vi "judgeExtremeType.vi"(9 "next":i8, 10 "current":i8, 11 "previous":i8) -> (0 "isExtreme?":bool, 3 "extreme Type":u8)   [LabVIEW 2016]
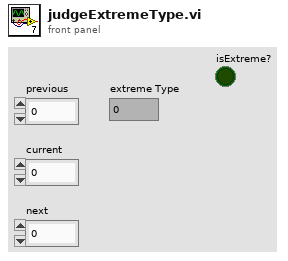
[diagram p1: front panel]
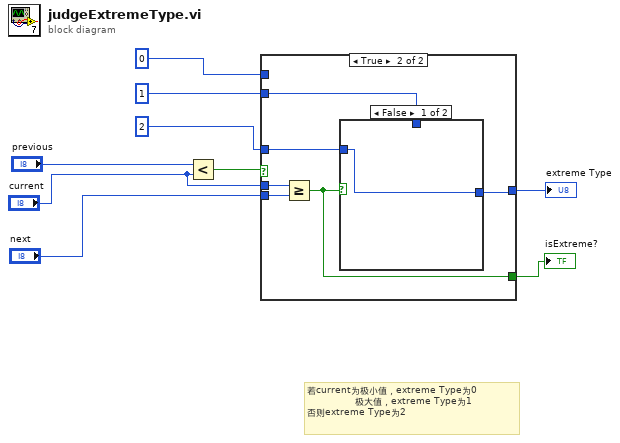
[diagram p0: block diagram]
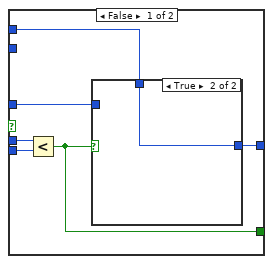
[diagram p2: hidden frame]
diagram:
  # "若current为极小值，extreme Type为0\n                极大值，extreme Type为1\n否则extreme Type为2"
  n1 = Less?(x="previous", y="current") -> (x < y?=w6:bool)
  n2 = case shown="True" w6 {
    tunnel: "current" -> [w15 w23]
    tunnel: "next" -> [w14 w22]
    tunnel: [w12 w19] -> w9
    tunnel: i16 1 -> [_ w21]
    tunnel: i16 0 -> [w13 _]
    tunnel: i16 2 -> [w11 w20]
    tunnel: [w10 w18] -> w1
    frame False {
      n3 = Less?(x=w15, y=w14) -> (x < y?=w10:bool)
      n4 = case shown="True" w10 {
        tunnel: [w16 w17] -> w12
        tunnel: w13 -> [_ w17]
        tunnel: w11 -> [w16 _]
        frame False {
        }
        frame True {
        }
      }
    }
    frame True {
      n5 = Greater Or Equal?(x=w23, y=w22) -> (x >= y?=w18:bool)
      n6 = case shown="False" w18 {
        tunnel: [w24 w25] -> w19
        tunnel: w21 -> [_ w25]
        tunnel: w20 -> [w24 _]
        frame False {
        }
        frame True {
        }
      }
    }
  }
  "extreme Type" <- w9
  "isExtreme?" <- w1
